vi "Tab Handler.vi"(0 "RunScreen Ref":refnum<vi>, 2 "Mode":T1(ring), 5 "Test Config Ref":refnum<vi>, 7 "Stand Config Ref":refnum<vi>) -> ()   [LabVIEW 2019]
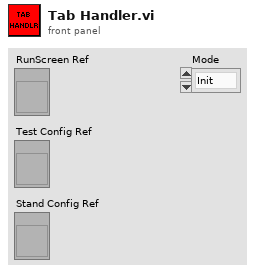
[diagram p1: front panel]
types:
  T1 = enum16{"Init", "Run Screen", "Test Config", "Stand Config", "Lock All", "Other Tab"}
  T2 = enum8{"Enabled", "Disabled", "Disabled and Grayed Out"}
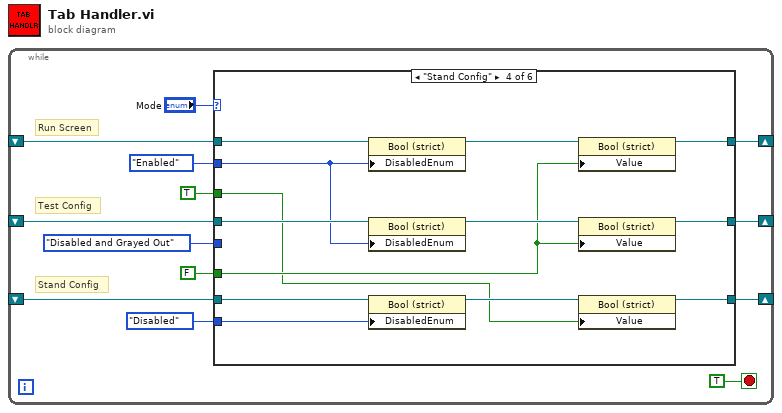
[diagram p0: block diagram]
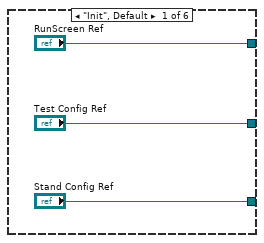
[diagram p2: hidden frame]
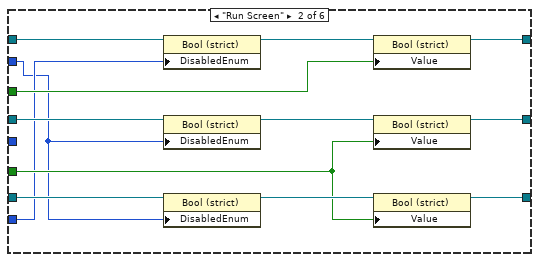
[diagram p3: hidden frame]
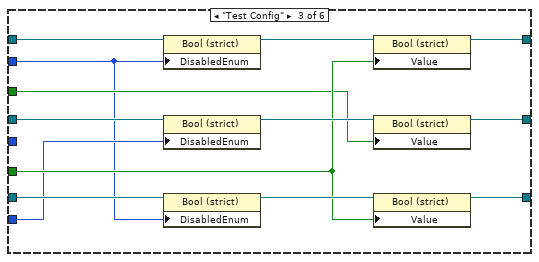
[diagram p4: hidden frame]
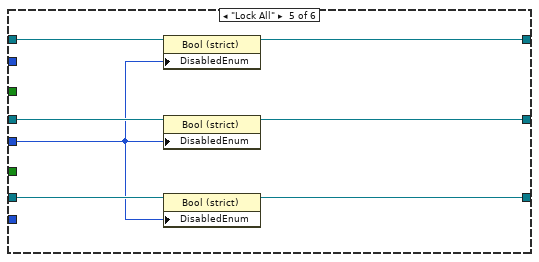
[diagram p5: hidden frame]
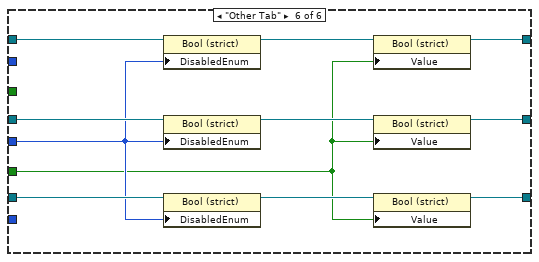
[diagram p6: hidden frame]
diagram:
  n1 = while {
    shift-right: [w11] -> _
    shift-left: _ -> [w8]
    shift-right: [w10] -> _
    shift-left: _ -> [w7]
    shift-right: [w9] -> _
    shift-left: _ -> [w6]
    stop <- TRUE stop-if-true
    # "Stand Config"
    # "Test Config"
    # "Run Screen"
    n2 = case shown="\"Stand Config\"" "Mode" {
      tunnel: ["RunScreen Ref" w22 w35 w48 w59 w66] -> w11
      tunnel: ["Test Config Ref" w23 w36 w49 w58 w67] -> w10
      tunnel: ["Stand Config Ref" w26 w39 w52 w57 w70] -> w9
      tunnel: w8 -> [_ w29 w42 w55 w62 w73]
      tunnel: w7 -> [_ w25 w38 w51 w60 w69]
      tunnel: w6 -> [_ w28 w41 w54 w61 w72]
      tunnel: T2."Enabled" ("Disabled") -> [_ w17 w30 w44 _ _]
      tunnel: T2."Disabled and Grayed Out" ("Disabled") -> [_ _ _ _ w56 w64]
      tunnel: TRUE -> [_ w20 w32 w45 _ _]
      tunnel: FALSE -> [_ w19 w33 w46 _ w63]
      tunnel: T2."Disabled" ("Disabled") -> [_ w18 w31 w43 _ _]
      frame "Init", Default {
      }
      frame "Run Screen" {
        n3 = property class="Bool (strict)"(reference=w29, "DisabledEnum"=w18) -> (reference out=w21:refnum<vi>)  [unwired: 1 in, 1 out]
        n4 = property class="Bool (strict)"(reference=w25, "DisabledEnum"=w17) -> (reference out=w24:refnum<vi>)  [unwired: 1 in, 1 out]
        n5 = property class="Bool (strict)"(reference=w28, "DisabledEnum"=w17) -> (reference out=w27:refnum<vi>)  [unwired: 1 in, 1 out]
        n6 = property class="Bool (strict)"(reference=w21, "Value"=w20) -> (reference out=w22:refnum<vi>)  [unwired: 1 in, 1 out]
        n7 = property class="Bool (strict)"(reference=w24, "Value"=w19) -> (reference out=w23:refnum<vi>)  [unwired: 1 in, 1 out]
        n8 = property class="Bool (strict)"(reference=w27, "Value"=w19) -> (reference out=w26:refnum<vi>)  [unwired: 1 in, 1 out]
      }
      frame "Test Config" {
        n9 = property class="Bool (strict)"(reference=w42, "DisabledEnum"=w30) -> (reference out=w34:refnum<vi>)  [unwired: 1 in, 1 out]
        n10 = property class="Bool (strict)"(reference=w38, "DisabledEnum"=w31) -> (reference out=w37:refnum<vi>)  [unwired: 1 in, 1 out]
        n11 = property class="Bool (strict)"(reference=w41, "DisabledEnum"=w30) -> (reference out=w40:refnum<vi>)  [unwired: 1 in, 1 out]
        n12 = property class="Bool (strict)"(reference=w34, "Value"=w33) -> (reference out=w35:refnum<vi>)  [unwired: 1 in, 1 out]
        n13 = property class="Bool (strict)"(reference=w37, "Value"=w32) -> (reference out=w36:refnum<vi>)  [unwired: 1 in, 1 out]
        n14 = property class="Bool (strict)"(reference=w40, "Value"=w33) -> (reference out=w39:refnum<vi>)  [unwired: 1 in, 1 out]
      }
      frame "Stand Config" {
        n15 = property class="Bool (strict)"(reference=w55, "DisabledEnum"=w44) -> (reference out=w47:refnum<vi>)  [unwired: 1 in, 1 out]
        n16 = property class="Bool (strict)"(reference=w51, "DisabledEnum"=w44) -> (reference out=w50:refnum<vi>)  [unwired: 1 in, 1 out]
        n17 = property class="Bool (strict)"(reference=w54, "DisabledEnum"=w43) -> (reference out=w53:refnum<vi>)  [unwired: 1 in, 1 out]
        n18 = property class="Bool (strict)"(reference=w47, "Value"=w46) -> (reference out=w48:refnum<vi>)  [unwired: 1 in, 1 out]
        n19 = property class="Bool (strict)"(reference=w50, "Value"=w46) -> (reference out=w49:refnum<vi>)  [unwired: 1 in, 1 out]
        n20 = property class="Bool (strict)"(reference=w53, "Value"=w45) -> (reference out=w52:refnum<vi>)  [unwired: 1 in, 1 out]
      }
      frame "Lock All" {
        n21 = property class="Bool (strict)"(reference=w62, "DisabledEnum"=w56) -> (reference out=w59:refnum<vi>)  [unwired: 1 in, 1 out]
        n22 = property class="Bool (strict)"(reference=w60, "DisabledEnum"=w56) -> (reference out=w58:refnum<vi>)  [unwired: 1 in, 1 out]
        n23 = property class="Bool (strict)"(reference=w61, "DisabledEnum"=w56) -> (reference out=w57:refnum<vi>)  [unwired: 1 in, 1 out]
      }
      frame "Other Tab" {
        n24 = property class="Bool (strict)"(reference=w73, "DisabledEnum"=w64) -> (reference out=w65:refnum<vi>)  [unwired: 1 in, 1 out]
        n25 = property class="Bool (strict)"(reference=w69, "DisabledEnum"=w64) -> (reference out=w68:refnum<vi>)  [unwired: 1 in, 1 out]
        n26 = property class="Bool (strict)"(reference=w72, "DisabledEnum"=w64) -> (reference out=w71:refnum<vi>)  [unwired: 1 in, 1 out]
        n27 = property class="Bool (strict)"(reference=w65, "Value"=w63) -> (reference out=w66:refnum<vi>)  [unwired: 1 in, 1 out]
        n28 = property class="Bool (strict)"(reference=w68, "Value"=w63) -> (reference out=w67:refnum<vi>)  [unwired: 1 in, 1 out]
        n29 = property class="Bool (strict)"(reference=w71, "Value"=w63) -> (reference out=w70:refnum<vi>)  [unwired: 1 in, 1 out]
      }
    }
  }
